vi "TimingFunctions_getUtcTimestamp.vi"() -> (0 "UTC-time":timestamp format="%^<%H:%M:%S%3u %p\n%d/%m/%Y>T")   [LabVIEW 2016]
doc: "Gibt den Timestamp in UTC aus.\n\n11.3.15 / sige"
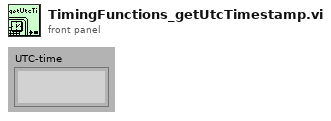
[diagram p1: front panel]
types:
  T1 = typedef "LVDateTimeRec.ctl" = cluster{"fractional second":dbl, "second":i32, "minute":i32, "hour":i32, "day of month":i32, "month":i32, "year":i32, "day of week":i32, "day of year":i32, "DST":i32}
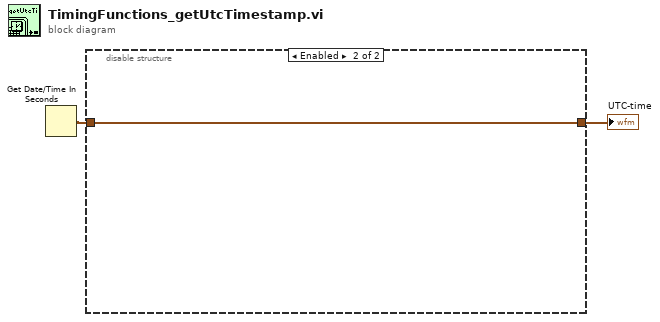
[diagram p0: block diagram]
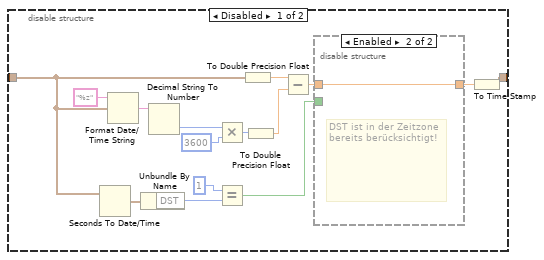
[diagram p2: hidden frame]
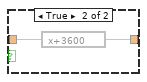
[diagram p4: hidden frame]
diagram:
  n1 = Get Date/Time In Seconds() -> (seconds since 1Jan1904=w1:timestamp)
  n2 = disable-structure shown="Enabled" {
    disable-tunnel: [w10 w25] -> w2
    disable-tunnel: w1 -> [w9 w25]
    frame Disabled {
      n3 = Seconds To Date/Time(time stamp (now)=w9) -> (date time rec=w8:T1)  [unwired: 1 in]
      n4 = Format Date/Time String(time format string (%c)="%z", seconds (now)=w9) -> (date/time string=w12:string)  [unwired: 1 out]
      n5 = Unbundle By Name(w8) -> ("DST"=w7:i32)
      n6 = Decimal String To Number(string=w12) -> (number=w11:i32)  [unwired: 3 out]
      n7 = Multiply(x=w11, y=3600) -> (x*y=w15:i32)
      n8 = Equal?(x=1, y=w7) -> (x = y?=w5:bool)
      n9 = To Double Precision Float(number=w9) -> (double precision float=w14:dbl)
      n10 = To Double Precision Float(number=w15) -> (double precision float=w13:dbl)
      n11 = Subtract(x=w14, y=w13) -> (x-y=w4:dbl)
      n12 = disable-structure shown="Enabled" {
        disable-tunnel: w5 -> [w20 _]
        disable-tunnel: w4 -> [w19 w24]
        disable-tunnel: [w18 w24] -> w3
        frame Disabled {
          n13 = case shown="False" w20 {
            tunnel: w19 -> [w21 w23]
            tunnel: [w21 w22] -> w18
            frame False {
            }
            frame True {
              n14 = expression code="x+3600"(w23) -> (w22:dbl)
            }
          }
        }
        frame Enabled {
          # "DST ist in der Zeitzone bereits berücksichtigt!"
        }
      }
      n15 = To Time Stamp(1:w3) -> (0:w10:timestamp)
    }
    frame Enabled {
    }
  }
  "UTC-time" <- w2
